vi "Parameters.vi"() -> ()   [LabVIEW 2016, in "NI-PCG Vehicle Model.lvlib"]
uses:
  NI-PCG Vehicle Model.lvlib
  Types/Engine Parameters.ctl
  Types/Transmission Parameters.ctl
  Types/Vehicle Parameters.ctl
panel:
  in  "Parameters":T4={"Engine Parameters"={"Ambient Parameters"={"Temperature (K)"=288.0, "Pressure (Pa)"=101325.01}, "Air Parameters"={"R (Ideal Gas Constant)"=287.05, "Molecular Weight"=28.964, "Cp (Specific Heat Constant)"=1005.0, "Density (kg/m^3)"=1.229, "Stoichiometric A/F Ratio"=14.7}, "Engine Geometry Parameters"={"Cylinder Volume (l)"=1.794, "J (Rotational Moment of Inertia)"=0.14, "Minimuim Engine Speed"=47.12385, "Maximum Engine Speed"=733.03766, "Intake Manifold Volume (l)"=3.588}, "Volumetric Efficiency Map"={"MAP"=[0.0, 0.0625, 0.125, 0.1875, 0.25, 0.3125, 0.375, 0.4375, 0.5, 0.5625, 0.625, 0.6875, 0.75, 0.8125, 0.875, 0.9375, 1.0], "RPM"=[200.0, 700.0, 1000.0, 1200.0, 1800.0, 2200.0, 2600.0, 3000.0, 3400.0, 3800.0, 4200.0, 4600.0, 5000.0, 5400.0, 5800.0, 6200.0], "Table"=[[0.001, 0.001, 0.001, 0.001, 0.001, 0.001, 0.001, 0.001, 0.001, 0.001, 0.001, 0.001, 0.001, 0.001, 0.001, 0.001], [0.002, 0.002, 0.002, 0.002, 0.002, 0.002, 0.002, 0.002, 0.002, 0.002, 0.002, 0.002, 0.002, 0.002, 0.002, 0.002], [0.003, 0.003, 0.003, 0.003, 0.003, 0.003, 0.003, 0.003, 0.003, 0.003, 0.003, 0.003, 0.003, 0.003, 0.003, 0.003], [0.004, 0.004, 0.004, 0.004, 0.004, 0.004, 0.004, 0.004, 0.004, 0.004, 0.004, 0.004, 0.004, 0.004, 0.004, 0.004], [0.392, 0.392, 0.436, 0.451, 0.505, 0.544, 0.515, 0.51, 0.515, 0.52, 0.52, 0.52, 0.52, 0.52, 0.52, 0.52], [0.402, 0.402, 0.446, 0.466, 0.534, 0.554, 0.564, 0.574, 0.603, 0.637, 0.647, 0.647, 0.647, 0.618, 0.574, 0.544], [0.417, 0.431, 0.466, 0.529, 0.554, 0.569, 0.618, 0.618, 0.627, 0.657, 0.657, 0.657, 0.657, 0.627, 0.608, 0.564], [0.446, 0.451, 0.485, 0.559, 0.603, 0.618, 0.657, 0.662, 0.667, 0.672, 0.672, 0.672, 0.672, 0.657, 0.618, 0.574], [0.461, 0.544, 0.578, 0.569, 0.613, 0.632, 0.652, 0.662, 0.681, 0.676, 0.676, 0.676, 0.676, 0.657, 0.627, 0.608], [0.51, 0.51, 0.52, 0.593, 0.618, 0.632, 0.642, 0.647, 0.657, 0.676, 0.681, 0.681, 0.681, 0.667, 0.632, 0.608], [0.52, 0.52, 0.539, 0.593, 0.627, 0.652, 0.657, 0.662, 0.676, 0.681, 0.681, 0.681, 0.681, 0.676, 0.637, 0.613], [0.559, 0.559, 0.544, 0.608, 0.642, 0.657, 0.662, 0.676, 0.681, 0.681, 0.686, 0.686, 0.686, 0.676, 0.647, 0.627], [0.583, 0.583, 0.564, 0.637, 0.647, 0.672, 0.676, 0.681, 0.681, 0.681, 0.686, 0.686, 0.686, 0.681, 0.662, 0.623], [0.618, 0.608, 0.632, 0.642, 0.672, 0.735, 0.691, 0.701, 0.725, 0.696, 0.681, 0.681, 0.676, 0.657, 0.632, 0.608], [0.657, 0.618, 0.652, 0.681, 0.691, 0.75, 0.804, 0.814, 0.848, 0.824, 0.824, 0.828, 0.828, 0.794, 0.789, 0.74], [0.681, 0.691, 0.667, 0.711, 0.73, 0.775, 0.833, 0.868, 0.873, 0.848, 0.838, 0.828, 0.828, 0.824, 0.794, 0.76], [0.681, 0.691, 0.667, 0.711, 0.73, 0.775, 0.833, 0.868, 0.873, 0.848, 0.838, 0.828, 0.828, 0.824, 0.794, 0.76]]}, "Fuel LHV (J/kg)"=42700000.0, "Combustion Efficiency Map"={"Spark Timing (deg BTDC))"=[0.0, 25.0, 50.0], "Engine Speed (RPM)"=[200.0, 6200.0], "Combustion Efficiency"=[[0.75, 0.75], [1.0, 1.0], [0.75, 0.75]]}, "Thermodynamic Efficiency"=0.4}, "Transmission Parameters"={"Final Drive Ratio"=2.655, "Transmission Gear Ratios"={"Gears"=[1.0, 2.0, 3.0, 4.0], "Gear Ratios"=[3.643, 2.008, 1.296, 0.892]}, "Torque Converter Map"={"Speed Ratio"=[0.0, 0.1, 0.2, 0.3, 0.4, 0.5, 0.6, 0.7, 0.8, 0.81, 0.82, 0.83, 0.84, 0.85, 0.86, 0.87, 0.88, 0.89, 0.9, 0.92, 0.94, 0.97], "K Factor"=[18.9894, 18.9341, 18.7683, 18.7407, 19.0033, 19.3902, 20.0674, 21.1178, 22.5137, 22.6933, 22.9559, 23.2047, 23.4949, 23.8681, 24.2274, 24.8079, 25.3607, 26.2314, 27.3094, 29.8247, 33.7774, 50.0], "Torque Ratio"=[2.232, 2.075, 1.975, 1.846, 1.72, 1.564, 1.409, 1.254, 1.096, 1.08, 1.061, 1.043, 1.028, 1.012, 1.002, 1.002, 1.001, 0.998, 0.997, 0.996, 0.995, 0.994]}, "Upshift Throttle"=[0.0, 25.0, 35.0, 50.0, 90.0, 100.0], "Downshift Throttle"=[0.0, 5.0, 40.0, 50.0, 90.0, 100.0], "Upshift Table"=[[10.0, 30.0, 50.0, 1000000.0], [10.0, 30.0, 50.0, 1000000.0], [15.0, 30.0, 50.0, 1000000.0], [23.0, 41.0, 60.0, 1000000.0], [40.0, 70.0, 100.0, 1000000.0], [40.0, 70.0, 100.0, 1000000.0]], "Downshift Table"=[[0.0, 5.0, 20.0, 35.0], [0.0, 5.0, 20.0, 35.0], [0.0, 5.0, 25.0, 40.0], [0.0, 5.0, 30.0, 50.0], [0.0, 30.0, 50.0, 80.0], [0.0, 30.0, 50.0, 80.0]], "Wait Time"=2}, "Vehicle Parameters"={"Vehicle Mass (kg)"=1133.98, "Vehicle Cd"=0.2, "Vehicle Frontal Area (m^2)"=2.384, "Wheel Radius (m)"=0.1778, "Wheel Rolling Resistance"=0.012}} {"Engine Parameters"."Engine Geometry Parameters"."Intake Manifold Volume (l)" format="%#_6p"}
  in  "ManualShiftEnable":bool
  in  "ManualShiftDown":bool
  in  "ManualShiftUp":bool
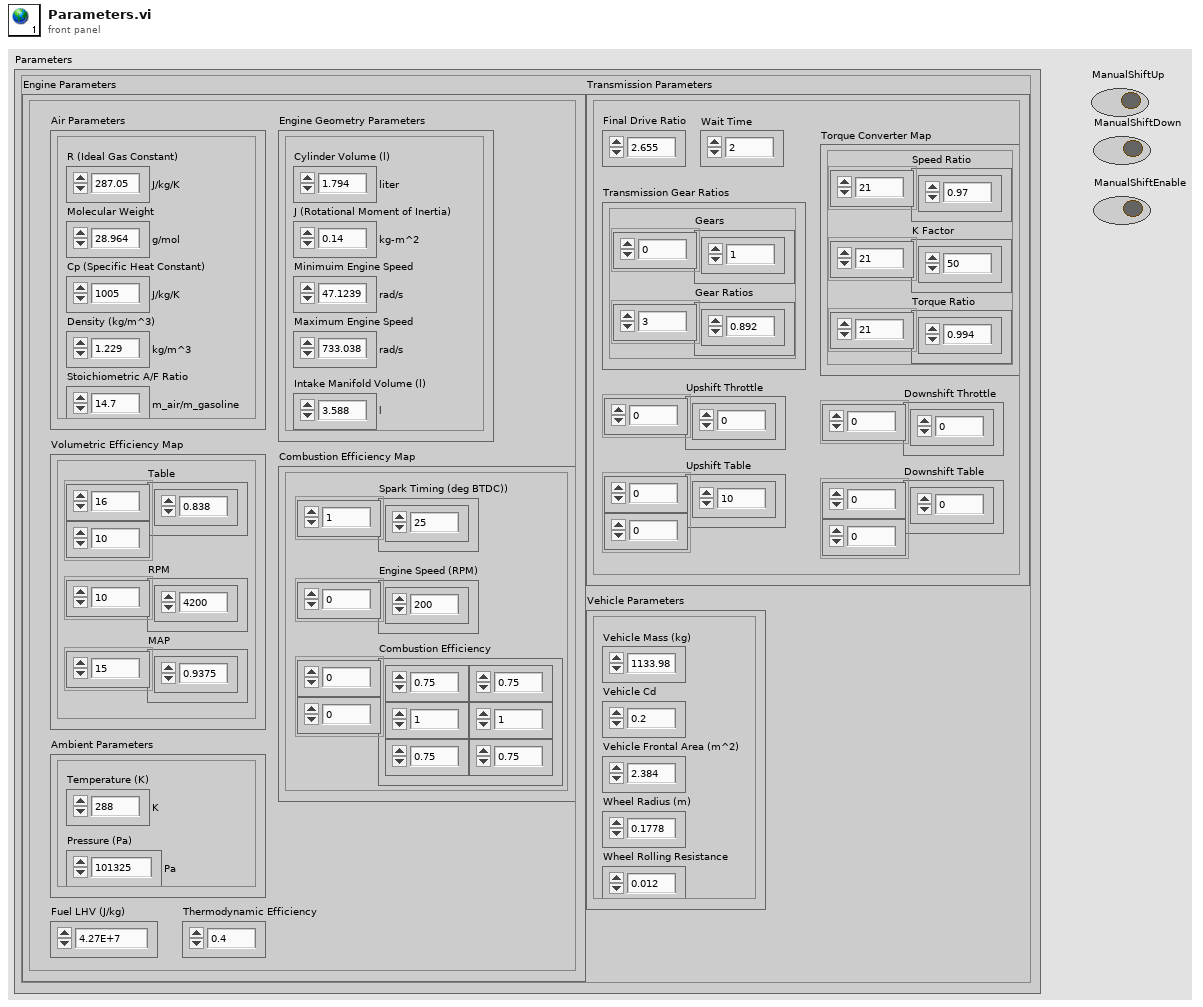
[diagram p1: front panel]
types:
  T1 = typedef "NI-PCG Vehicle Model.lvlib/Engine Parameters.ctl" = cluster{"Ambient Parameters":cluster{"Temperature (K)":sgl, "Pressure (Pa)":sgl}, "Air Parameters":cluster{"R (Ideal Gas Constant)":sgl, "Molecular Weight":sgl, "Cp (Specific Heat Constant)":sgl, "Density (kg/m^3)":sgl, "Stoichiometric A/F Ratio":sgl}, "Engine Geometry Parameters":cluster{"Cylinder Volume (l)":sgl, "J (Rotational Moment of Inertia)":sgl, "Minimuim Engine Speed":sgl, "Maximum Engine Speed":sgl, "Intake Manifold Volume (l)":sgl}, "Volumetric Efficiency Map":cluster{"MAP":sgl[], "RPM":sgl[], "Table":sgl[][]}, "Fuel LHV (J/kg)":sgl, "Combustion Efficiency Map":cluster{"Spark Timing (deg BTDC))":sgl[], "Engine Speed (RPM)":sgl[], "Combustion Efficiency":sgl[][]}, "Thermodynamic Efficiency":sgl}
  T2 = typedef "NI-PCG Vehicle Model.lvlib/Transmission Parameters.ctl" = cluster{"Final Drive Ratio":sgl, "Transmission Gear Ratios":cluster{"Gears":sgl[], "Gear Ratios":sgl[]}, "Torque Converter Map":cluster{"Speed Ratio":sgl[], "K Factor":sgl[], "Torque Ratio":sgl[]}, "Upshift Throttle":sgl[], "Downshift Throttle":sgl[], "Upshift Table":sgl[][], "Downshift Table":sgl[][], "Wait Time":u8}
  T3 = typedef "NI-PCG Vehicle Model.lvlib/Vehicle Parameters.ctl" = cluster{"Vehicle Mass (kg)":sgl, "Vehicle Cd":sgl, "Vehicle Frontal Area (m^2)":sgl, "Wheel Radius (m)":sgl, "Wheel Rolling Resistance":sgl}
  T4 = cluster{"Engine Parameters":T1, "Transmission Parameters":T2, "Vehicle Parameters":T3}
diagram:
